vi "Software package Integrity Tool.vi"() -> ()   [LabVIEW 2010]
uses:
  SIT_Data.ctl
  package/VIE.Module.Queued Message Handler.enqueue.State.PolyChild.QueuedMessageHandler.vi
  package/VIE.Module.Queued Message Handler.[enqueue].State.PolyChild.QueuedMessageHandler.vi
  <vilib>/Utility/config.llb/Read Key (String).vi
  package/Remove Duplicates from 1D Array (Path)__ogtk.vi
  package/VIE.Module.Queued Message Handler.QueuedMessageHandler.dqGOOPClass.lvlib
  <vilib>/Utility/config.llb/NI_LVConfig.lvlib
panel:
  out "File list not ok":string
  out "Package not ok":bool
  in  "Color Box":u32(colorbox)
  out "File List 2":i32[](listbox)
  out "Active Row:Cell Background Color":u32
  in  "chk package integrity":bool
  out "Error Out":errorcluster
  in  "Exit":bool
  in  "Add Package Integrity File":bool
  in  "Delete Package Integrity File":bool
  in  "Package Integrity Files":i32(listbox)
  in  "System Integrity File Path":path
  in  "Save System Integrity File":bool
  in  "User Name":string
  in  "Purpose":string
  in  "Package Revision":string
  in  "Package ID":string
  in  "Package Integrity File Path":path
  in  "Undo":bool
  in  "Save Package Integrity File":bool
  in  "Remove Selected Files":bool
  in  "Add VI Hierarchy":bool
  in  "Recursive":bool
  in  "Add Directory":bool
  in  "Add File":bool
  out "Selection Log":string
  in  "File List":i32[](listbox)
  in  "error in (no error)":errorcluster
  out "error out":errorcluster
  out "CVT (out)":T1
  # "Use the CVT as a data bus for data that is\nto be accesed outside of the VI.  It can be\nused for data passed around  inside the state\nmachine too, and all local data can be selectively\npurged from the CVT in the \"system.Exit\" state."
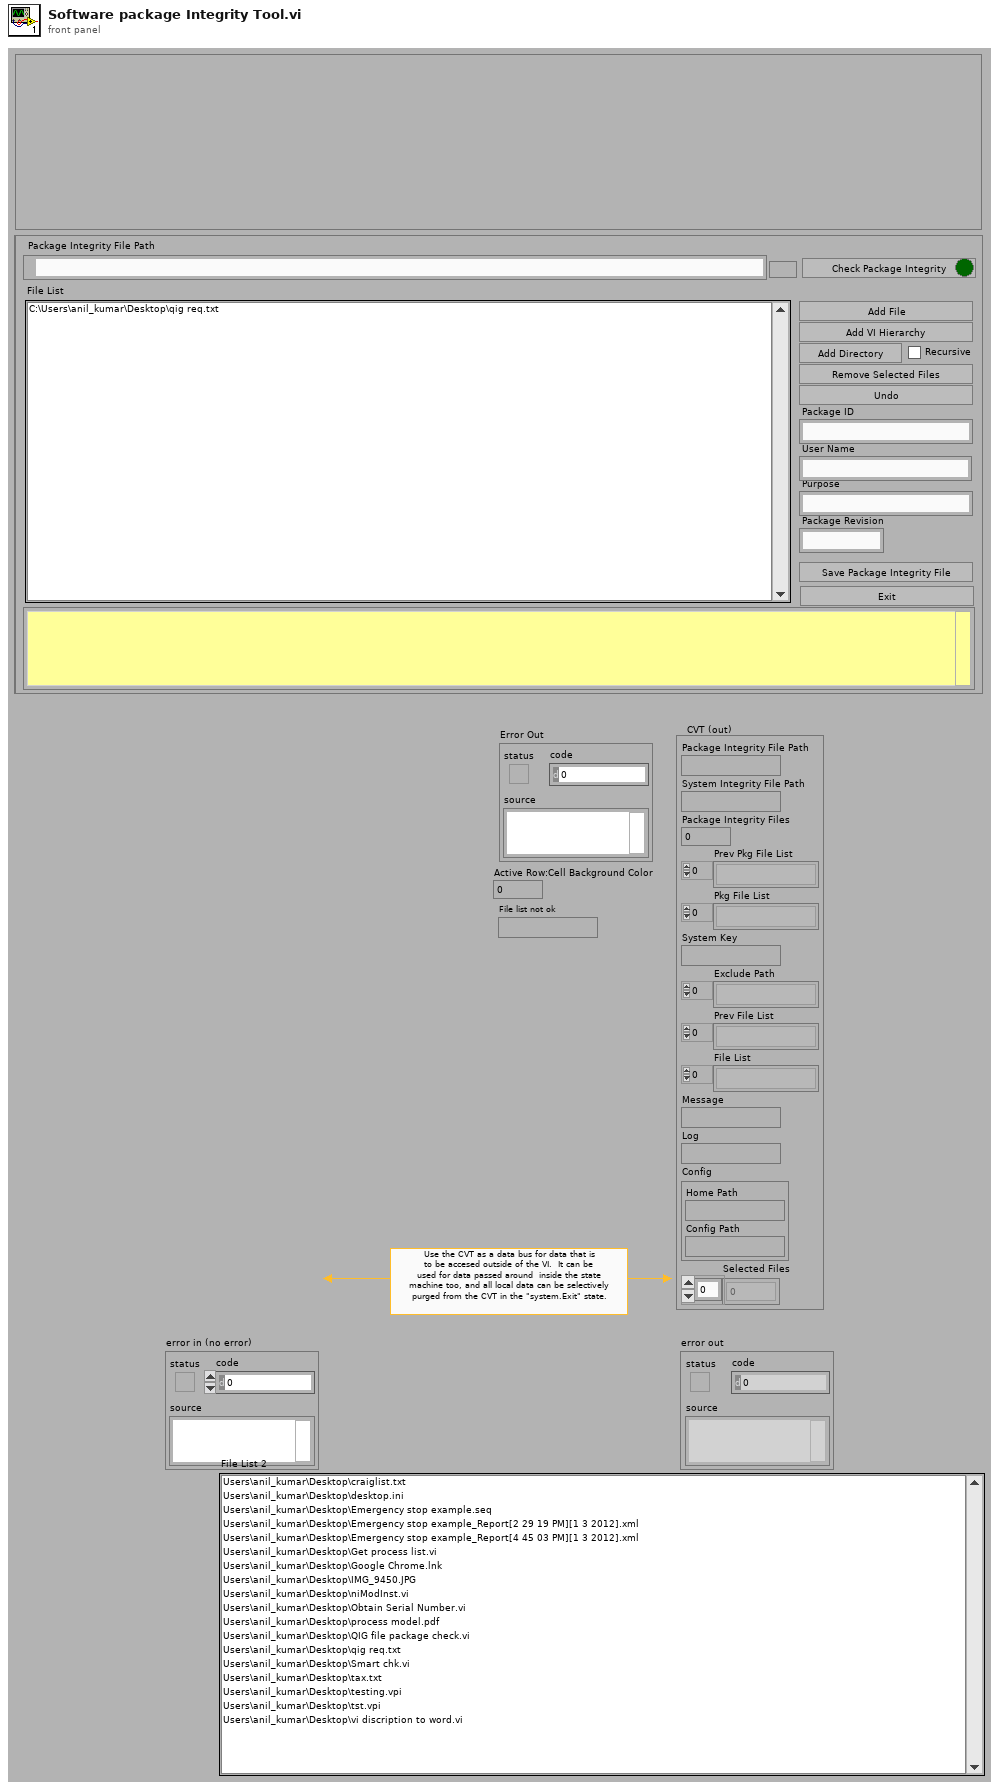
[diagram p1: front panel]
types:
  T1 = typedef "SIT_Data.ctl" = cluster{"Package Integrity File Path":path, "System Integrity File Path":path, "Package Integrity Files":i32, "Prev Pkg File List":path[], "Pkg File List":path[], "System Key":string, "Exclude Path":path[], "Prev File List":path[], "File List":path[], "Message":string, "Log":string, "Config":cluster{"Home Path":path, "Config Path":path}, "Selected Files":i32[]}
  T2 = typedef "VIE.Module.Queued Message Handler.QueuedMessageHandler.dqGOOPClass.lvlib/VIE.Module.Queued Message Handler.dqClass_ObjectReference.ctl" = refnum<k1>
  T3 = typedef "NI_LVConfig.lvlib/Config Data RefNum.ctl" = refnum<k1>
  T4 = enum32{"existing file", "new file", "new or existing file", "existing dir", "new dir", "new or existing dir", "existing file (use LLBs)", "new file (use LLBs)", "new or existing file (use LLBs)", "new or existing file or directory (use LLBs)", "existing dir (use LLBs)", "new dir (use LLBs)", "new or existing dir (use LLBs)", "existing file or dir", "new file or dir", "new or existing file or dir", "existing file or dir (use LLBs)", "new file or dir (use LLBs)"}
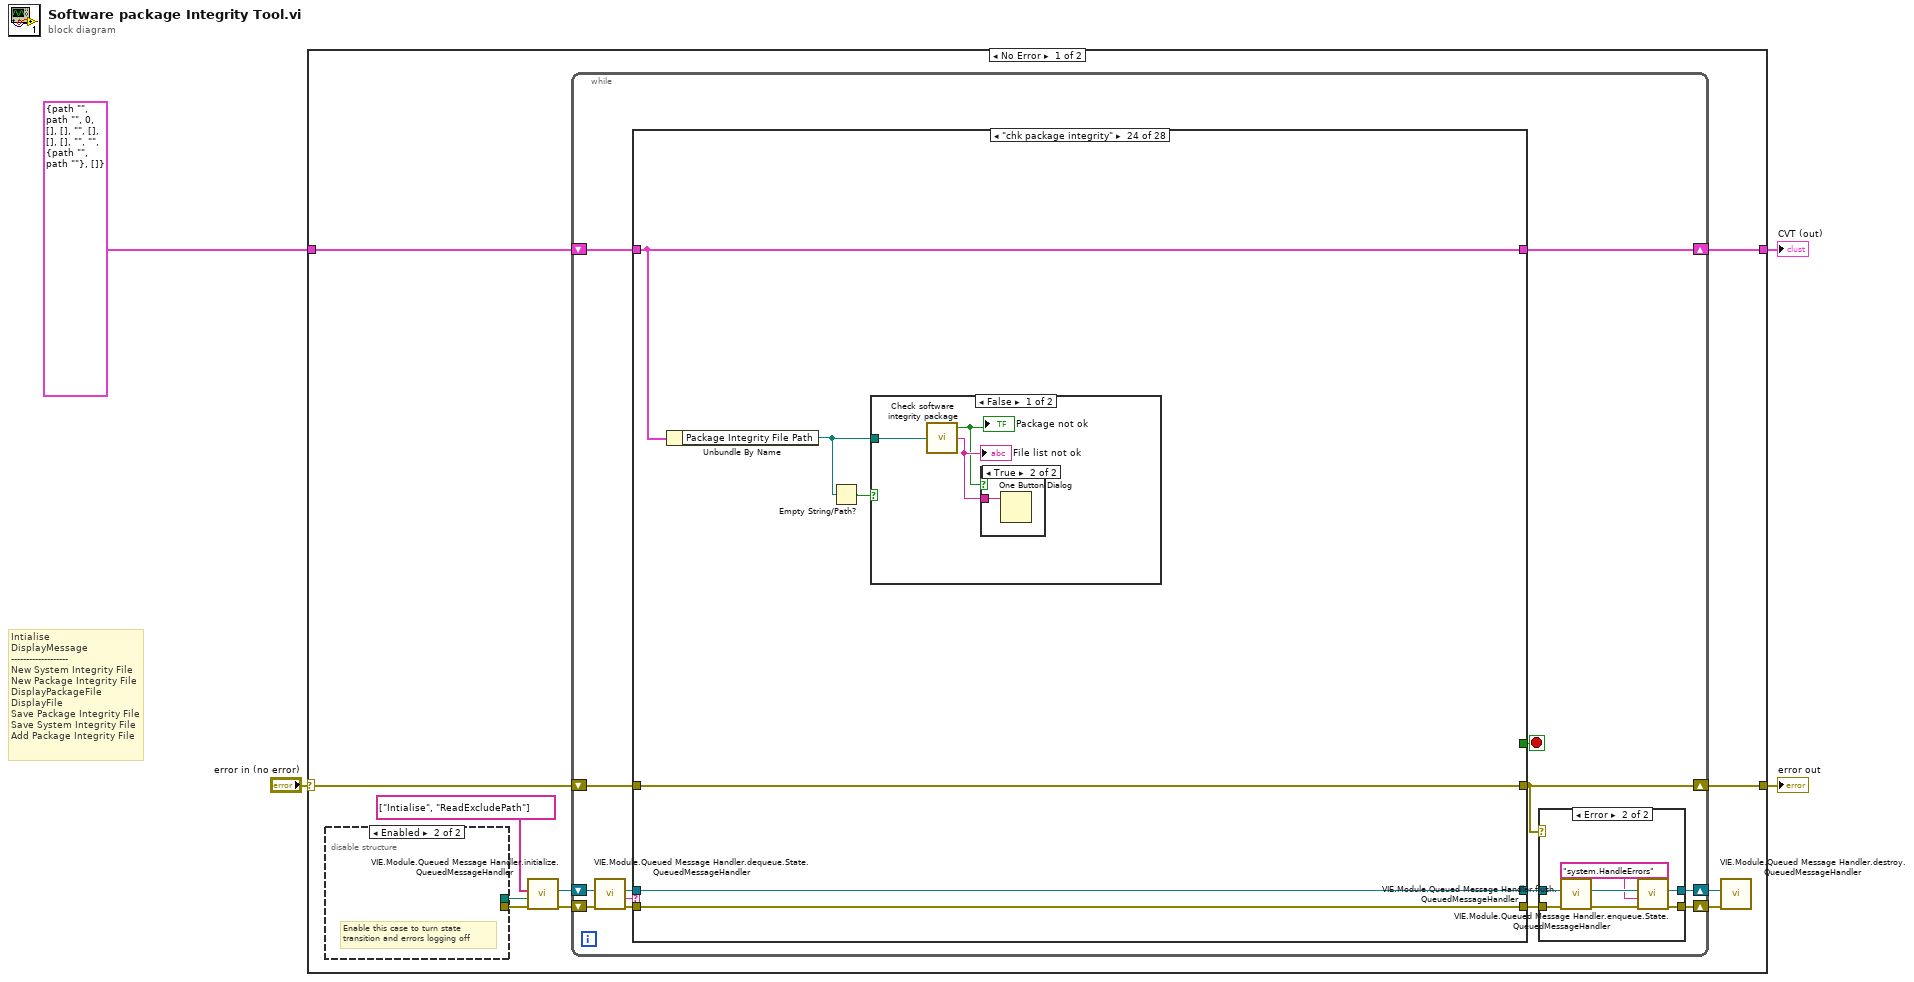
[diagram p0: block diagram]
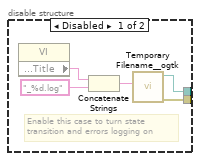
[diagram p2: hidden frame]
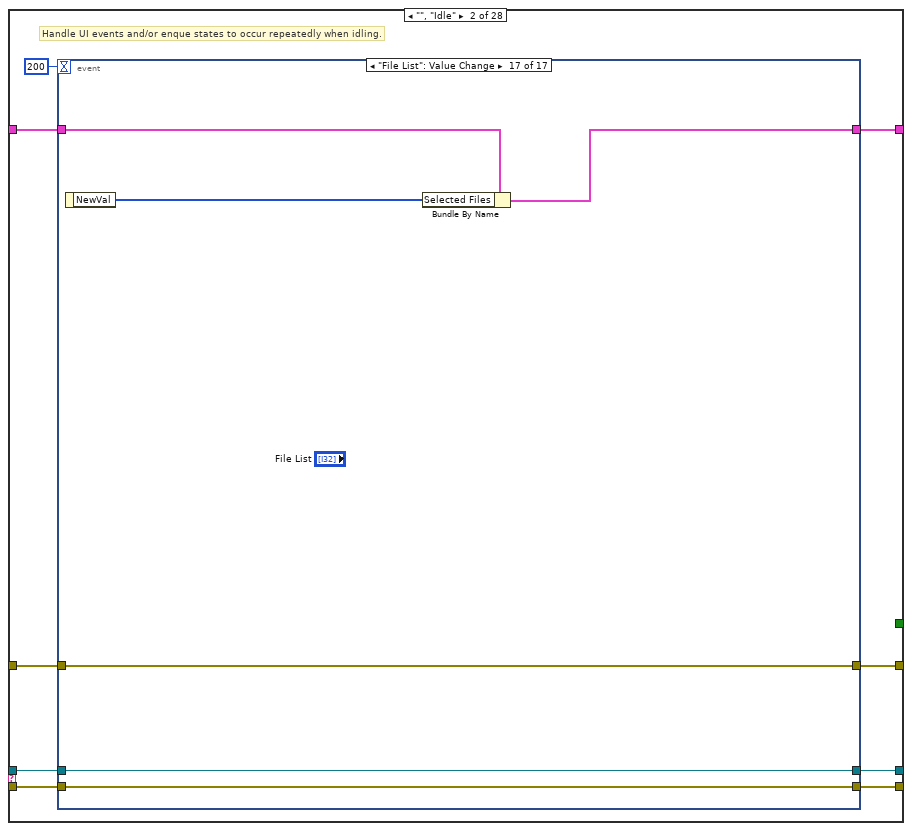
[diagram p5: hidden frame]
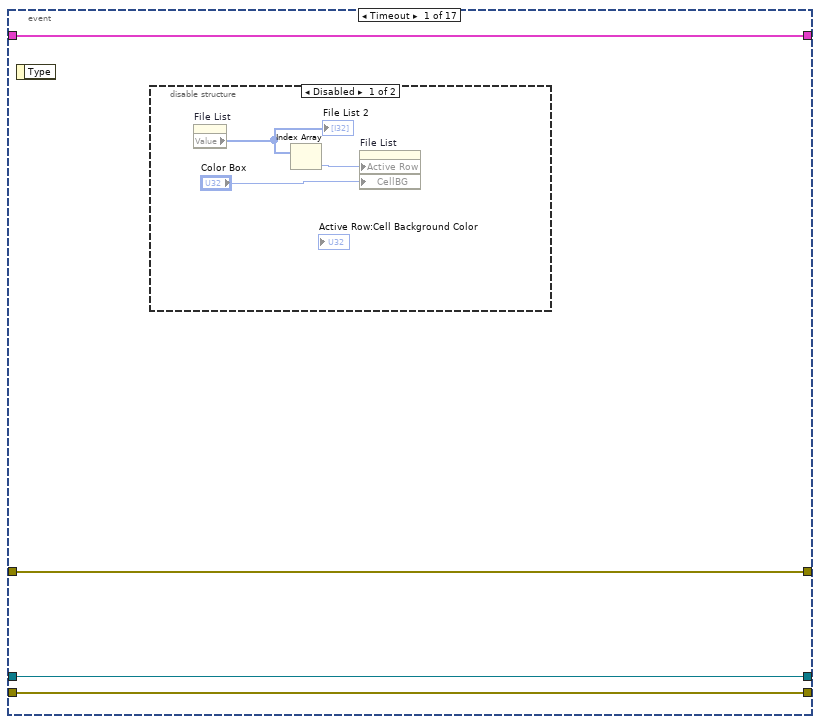
[diagram p6: hidden frame]
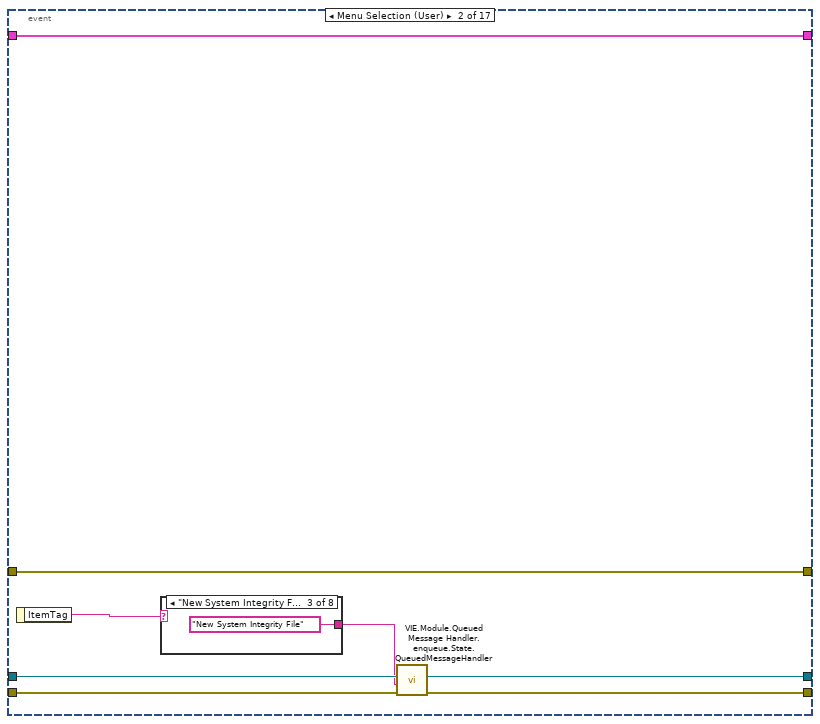
[diagram p8: hidden frame]
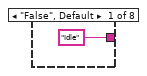
[diagram p9: hidden frame]
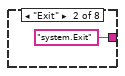
[diagram p10: hidden frame]
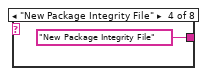
[diagram p11: hidden frame]
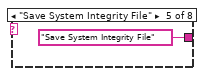
[diagram p12: hidden frame]
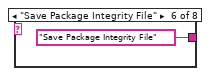
[diagram p13: hidden frame]
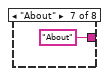
[diagram p14: hidden frame]
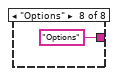
[diagram p15: hidden frame]
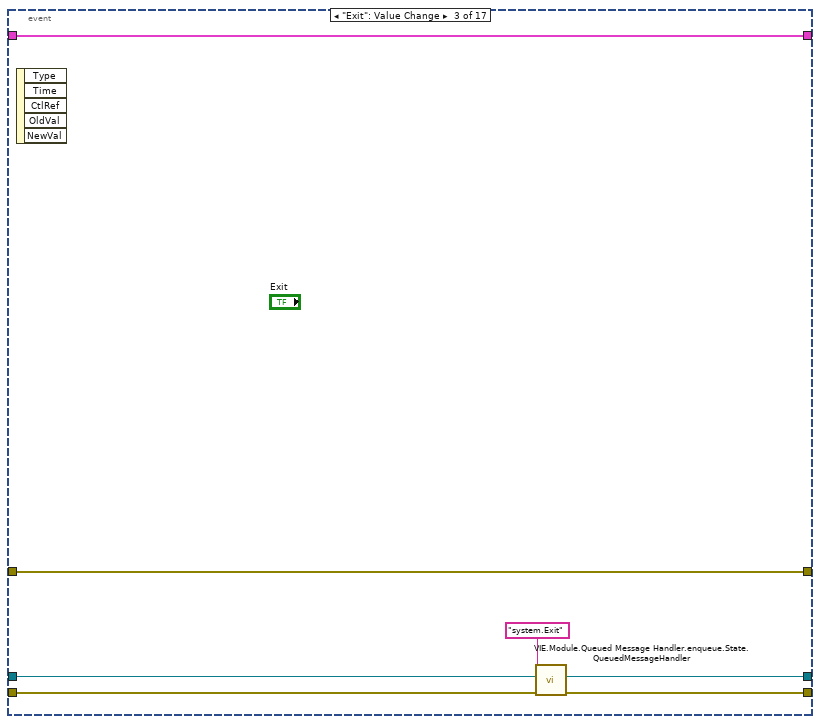
[diagram p16: hidden frame]
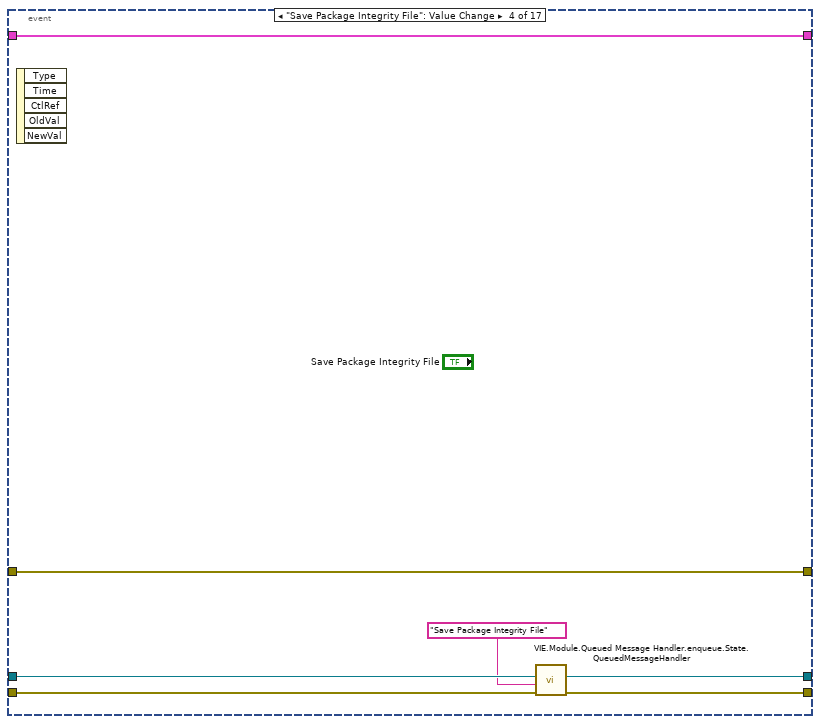
[diagram p17: hidden frame]
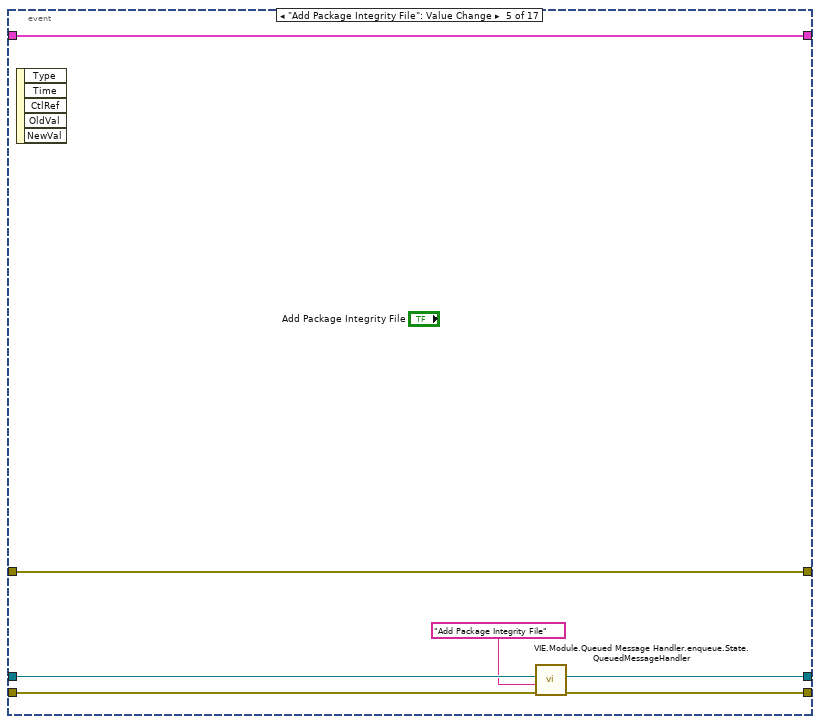
[diagram p18: hidden frame]
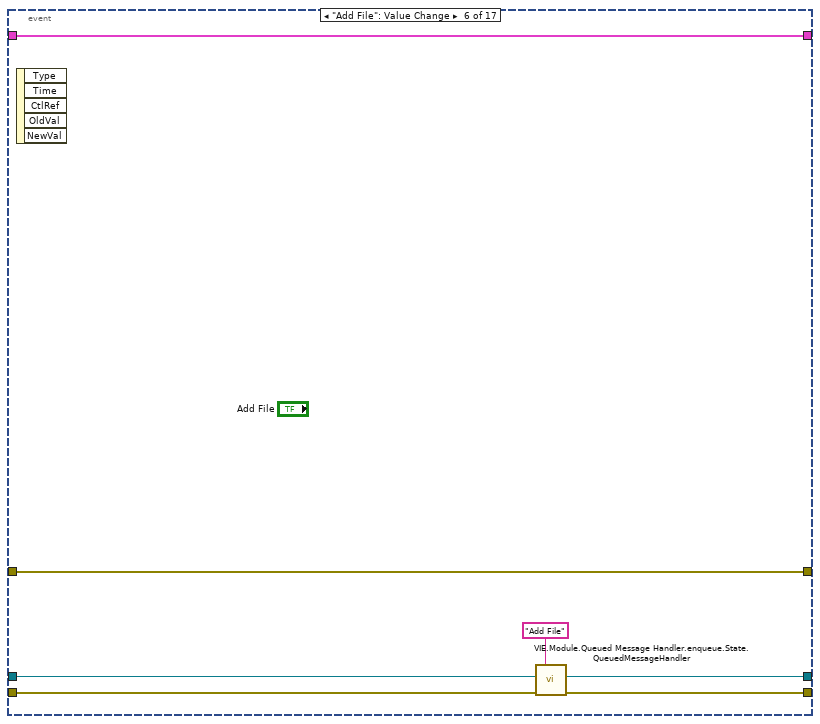
[diagram p19: hidden frame]
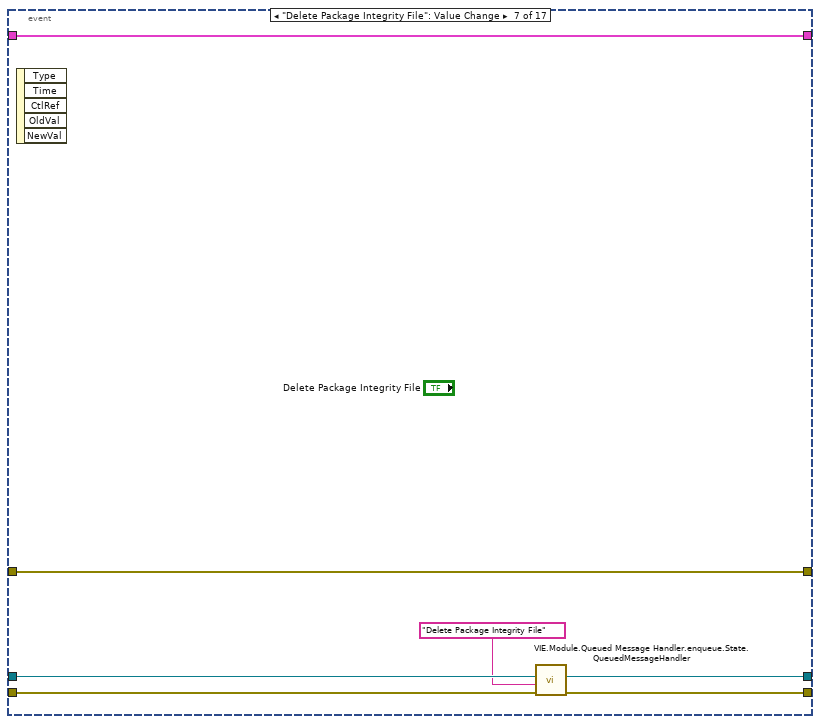
[diagram p20: hidden frame]
diagram:
  # "Intialise\nDisplayMessage\n-------------------\nNew System Integrity File\nNew Package Integrity File\nDisplayPackageFile\nDisplayFile\nSave Package Integrity File\nSave System Integrity File\nAdd Package Integrity File"
  n1 = case shown="No Error" "error in (no error)" {
    selector: "error in (no error)" -> [w8 w754]
    tunnel: [w7 w754] -> w2
    tunnel: T1 {"Package Integrity File Path"=path "", "System Integrity File Path"=path "", "Package Integrity Files"=0, "Prev Pkg File List"=[], "Pkg File List"=[], "System Key"="", "Exclude Path"=[], "Prev File List"=[], "File List"=[], "Message"="", "Log"="", "Config"={"Home Path"=path "", "Config Path"=path ""}, "Selected Files"=[]} ("CVT (in)") -> [w5 w753]
    tunnel: [w9 w753] -> w4
    frame No Error {
      n2 = disable-structure shown="Enabled" {
        disable-tunnel: [w17 _] -> w11
        disable-tunnel: [w16 _] -> w10
        frame Disabled {
          # "Enable this case to turn state\ntransition and errors logging on"
          n3 = property class="VI"() -> ("Front Panel.Title"=w18:string)  [unwired: 2 in, 2 out]
          n4 = Concatenate Strings(w18, "_%d.log" ("string")) -> (w20:string)
          n5 = call <userlib>:"Temporary Filename__ogtk.vi"("pattern (lvtemp%d.tmp)"=w20) -> ("error out"=w17:errorcluster, "file in tmp dir"=w16:path)  [unwired: 5 in]
        }
        frame Enabled {
          # "Enable this case to turn state\ntransition and errors logging off"
        }
      }
      n6 = call "VIE.Module.Queued Message Handler.initialize.QueuedMessageHandler.vi"("error in (no error)"=w11, "State Queue Log FilePath (\"\" = Do Not Log)"=w10, "Initial State Queue (empty)"=string[] ["Intialise", "ReadExcludePath"] ("Initial State Queue")) -> ("error out"=w15:errorcluster, "QueuedMessageHandler.dqGOOPClass (out)"=w12:T2)  [unwired: 7 in]
      n7 = while {
        shift-right: [w23] -> w14
        shift-left: w15 -> [w31]
        shift-right: [w28] -> w9
        shift-left: w5 -> [w29]
        shift-right: [w26] -> w7
        shift-left: w8 -> [w27]
        shift-right: [w22] -> w13
        shift-left: w12 -> [w34]
        stop <- w21 stop-if-true
        n8 = call "VIE.Module.Queued Message Handler.dequeue.State.QueuedMessageHandler.vi"("error in (no error)"=w31, "QueuedMessageHandler.dqGOOPClass (in)"=w34) -> ("error out"=w32:errorcluster, "State Dequeued"=w30:string, "QueuedMessageHandler.dqGOOPClass (out)"=w33:T2)  [unwired: 7 in]
        n9 = case shown="\"chk package integrity\"" w30 {
          selector: w30 -> [_ _ _ _ _ _ _ _ _ _ _ _ _ _ _ _ _ _ _ _ _ _ _ _ _ w714 _ _]
          tunnel: w32 -> [w44 w54 w203 w210 w231 w236 w265 w271 w277 w293 w308 w349 w360 w388 w410 w462 w479 w512 w542 w575 w630 w645 w655 w701 w708 w713 w731 w749]
          tunnel: [w44 w49 w200 w210 w231 w235 w263 w270 w277 w291 w306 w347 w359 w387 w409 w461 w478 w511 w541 w574 w629 w644 w654 w701 w708 w713 w722 w749] -> w25
          tunnel: w33 -> [w45 w53 w202 w211 w232 w234 w266 w269 w278 w294 w309 w350 w358 w386 w412 w460 w477 w510 w540 w573 w628 w643 w653 w702 w709 w712 w732 w750]
          tunnel: [w45 w50 w201 w211 w232 w233 w264 w268 w278 w292 w307 w348 w357 w385 w411 w459 w476 w509 w539 w572 w627 w642 w652 w702 w709 w712 w723 w750] -> w24
          tunnel: w29 -> [w47 w56 w207 w213 w222 w242 w267 w274 w280 w287 w300 w339 w366 w391 w419 w453 w471 w504 w536 w569 w626 w641 w659 w700 w711 w721 w735 w748]
          tunnel: [w47 w52 w206 w217 w221 w241 w267 w274 w280 w286 w304 w338 w365 w390 w418 w452 w470 w503 w535 w568 w625 w640 w658 w700 w711 w721 w735 w748] -> w28
          tunnel: w27 -> [w46 w55 w208 w212 w230 w243 w261 w275 w279 w289 w302 w345 w371 w399 w417 _ w469 w502 w534 w567 w624 w639 w674 w703 w710 w716 w733 w751]
          tunnel: [w46 w51 w194 w214 w230 w243 w261 w275 w279 w289 w301 w345 w371 w399 w416 w449 w468 w501 w533 w566 w624 w639 w674 w703 w710 w715 w726 w751] -> w26
          tunnel: [_ _ _ _ _ _ _ _ _ _ _ _ _ _ _ _ _ _ _ _ _ _ _ _ _ _ _ TRUE] -> w21
          frame "---- Custom States --------------------------" {
            # "Do not put any code in here - this is a case divider, and is not a valid state, so any code here will not be executed."
          }
          frame "", "Idle" {
            # "Handle UI events and/or enque states to occur repeatedly when idling."
            n10 = event shown="[16] \"File List\": Value Change" {
              selector: _ -> [_ _ _ _ _ _ _ _ _ _ _ _ _ _ _ _ _]
              dyn-events: _ -> [_ _ _ _ _ _ _ _ _ _ _ _ _ _ _ _ _]
              timeout: 200 -> [_ _ _ _ _ _ _ _ _ _ _ _ _ _ _ _ _]
              tunnel: w56 -> [w60 w71 w86 w93 w100 w107 w114 w121 w128 w135 w142 w149 w152 w162 w171 w185 w189]
              tunnel: w55 -> [w57 w70 w85 w92 w99 w106 w113 w120 w127 w134 w141 w148 w158 w169 w178 w184 w191]
              tunnel: w54 -> [w58 w69 w84 w91 w98 w105 w112 w119 w126 w133 w140 w147 w157 w168 w177 w181 w186]
              tunnel: w53 -> [w59 w67 w82 w89 w96 w103 w110 w117 w124 w131 w138 w145 w155 w166 w175 w182 w187]
              tunnel: [w60 w71 w86 w93 w100 w107 w114 w121 w128 w135 w142 w149 w151 w163 w172 w185 w190] -> w52
              tunnel: [w57 w70 w85 w92 w99 w106 w113 w120 w127 w134 w141 w148 w158 w169 w178 w184 w191] -> w51
              tunnel: [w59 w66 w81 w88 w95 w102 w109 w116 w123 w130 w137 w144 w154 w165 w174 w180 w187] -> w50
              tunnel: [w58 w68 w83 w90 w97 w104 w111 w118 w125 w132 w139 w146 w156 w167 w176 w179 w186] -> w49
              event Timeout {
                n11 = event-data() -> ()  [unwired: 1 in, 1 out]
                n12 = disable-structure shown="Disabled" {
                  frame Disabled {
                    n13 = property on="File List" class="LstBox (strict)"() -> ("Value"=w63:i32[])  [unwired: 2 in, 2 out]
                    "File List 2" <- w63
                    n14 = Index Array(array=w63) -> (element=w62:i32)  [unwired: 1 in]
                    n15 = property on="File List" class="LstBox (strict)"("Active Row"=w62, "CellBG"="Color Box") -> ()  [unwired: 2 in, 2 out]
                  }
                  frame Enabled {
                  }
                }
              }
              event Menu Selection (User) {
                n16 = event-data() -> ("ItemTag"=w65:string)  [unwired: 1 in]
                n17 = case shown="\"New System Integrity File\"" w65 {
                  tunnel: ["Idle" ("ItemTag") "system.Exit" ("ItemTag") "New System Integrity File" ("ItemTag") "New Package Integrity File" ("ItemTag") "Save System Integrity File" ("ItemTag") "Save Package Integrity File" ("ItemTag") "About" ("ItemTag") "Options" ("ItemTag")] -> w64
                  frame "False", Default {
                  }
                  frame "Exit" {
                  }
                  frame "New System Integrity File" {
                  }
                  frame "New Package Integrity File" {
                  }
                  frame "Save System Integrity File" {
                  }
                  frame "Save Package Integrity File" {
                  }
                  frame "About" {
                  }
                  frame "Options" {
                  }
                }
                n18 = call-poly "VIE.Module.Queued Message Handler.enqueue.State.QueuedMessageHandler.vi"("error in (no error)"=w69, "State to Enqueue"=w64, "QueuedMessageHandler.dqGOOPClass (in)"=w67) -> ("error out"=w68:errorcluster, "QueuedMessageHandler.dqGOOPClass (out)"=w66:T2)  [unwired: 7 in]
              }
              event "Exit": Value Change {
                n19 = event-data() -> ()  [unwired: 1 in, 5 out]
                n20 = call-poly "VIE.Module.Queued Message Handler.enqueue.State.QueuedMessageHandler.vi"("error in (no error)"=w84, "State to Enqueue"="system.Exit", "QueuedMessageHandler.dqGOOPClass (in)"=w82) -> ("error out"=w83:errorcluster, "QueuedMessageHandler.dqGOOPClass (out)"=w81:T2)  [unwired: 7 in]
              }
              event "Save Package Integrity File": Value Change {
                n21 = event-data() -> ()  [unwired: 1 in, 5 out]
                n22 = call-poly "VIE.Module.Queued Message Handler.enqueue.State.QueuedMessageHandler.vi"("error in (no error)"=w91, "State to Enqueue"="Save Package Integrity File", "QueuedMessageHandler.dqGOOPClass (in)"=w89) -> ("error out"=w90:errorcluster, "QueuedMessageHandler.dqGOOPClass (out)"=w88:T2)  [unwired: 7 in]
              }
              event "Add Package Integrity File": Value Change {
                n23 = event-data() -> ()  [unwired: 1 in, 5 out]
                n24 = call-poly "VIE.Module.Queued Message Handler.enqueue.State.QueuedMessageHandler.vi"("error in (no error)"=w98, "State to Enqueue"="Add Package Integrity File", "QueuedMessageHandler.dqGOOPClass (in)"=w96) -> ("error out"=w97:errorcluster, "QueuedMessageHandler.dqGOOPClass (out)"=w95:T2)  [unwired: 7 in]
              }
              event "Add File": Value Change {
                n25 = event-data() -> ()  [unwired: 1 in, 5 out]
                n26 = call-poly "VIE.Module.Queued Message Handler.enqueue.State.QueuedMessageHandler.vi"("error in (no error)"=w105, "State to Enqueue"="Add File", "QueuedMessageHandler.dqGOOPClass (in)"=w103) -> ("error out"=w104:errorcluster, "QueuedMessageHandler.dqGOOPClass (out)"=w102:T2)  [unwired: 7 in]
              }
              event "Delete Package Integrity File": Value Change {
                n27 = event-data() -> ()  [unwired: 1 in, 5 out]
                n28 = call-poly "VIE.Module.Queued Message Handler.enqueue.State.QueuedMessageHandler.vi"("error in (no error)"=w112, "State to Enqueue"="Delete Package Integrity File", "QueuedMessageHandler.dqGOOPClass (in)"=w110) -> ("error out"=w111:errorcluster, "QueuedMessageHandler.dqGOOPClass (out)"=w109:T2)  [unwired: 7 in]
              }
              event "Remove Selected Files": Value Change {
                n29 = event-data() -> ()  [unwired: 1 in, 5 out]
                n30 = call-poly "VIE.Module.Queued Message Handler.enqueue.State.QueuedMessageHandler.vi"("error in (no error)"=w119, "State to Enqueue"="Remove Selected Files", "QueuedMessageHandler.dqGOOPClass (in)"=w117) -> ("error out"=w118:errorcluster, "QueuedMessageHandler.dqGOOPClass (out)"=w116:T2)  [unwired: 7 in]
              }
              event "Add Directory": Value Change {
                n31 = event-data() -> ()  [unwired: 1 in, 5 out]
                n32 = call-poly "VIE.Module.Queued Message Handler.enqueue.State.QueuedMessageHandler.vi"("error in (no error)"=w126, "State to Enqueue"="Add Directory", "QueuedMessageHandler.dqGOOPClass (in)"=w124) -> ("error out"=w125:errorcluster, "QueuedMessageHandler.dqGOOPClass (out)"=w123:T2)  [unwired: 7 in]
              }
              event "Add VI Hierarchy": Value Change {
                n33 = event-data() -> ()  [unwired: 1 in, 5 out]
                n34 = call-poly "VIE.Module.Queued Message Handler.enqueue.State.QueuedMessageHandler.vi"("error in (no error)"=w133, "State to Enqueue"="Add VI Hierarchy", "QueuedMessageHandler.dqGOOPClass (in)"=w131) -> ("error out"=w132:errorcluster, "QueuedMessageHandler.dqGOOPClass (out)"=w130:T2)  [unwired: 7 in]
              }
              event "Undo": Value Change {
                n35 = event-data() -> ()  [unwired: 1 in, 5 out]
                n36 = call-poly "VIE.Module.Queued Message Handler.enqueue.State.QueuedMessageHandler.vi"("error in (no error)"=w140, "State to Enqueue"="Undo", "QueuedMessageHandler.dqGOOPClass (in)"=w138) -> ("error out"=w139:errorcluster, "QueuedMessageHandler.dqGOOPClass (out)"=w137:T2)  [unwired: 7 in]
              }
              event "Save System Integrity File": Value Change {
                n37 = event-data() -> ()  [unwired: 1 in, 5 out]
                n38 = call-poly "VIE.Module.Queued Message Handler.enqueue.State.QueuedMessageHandler.vi"("error in (no error)"=w147, "State to Enqueue"="Save System Integrity File", "QueuedMessageHandler.dqGOOPClass (in)"=w145) -> ("error out"=w146:errorcluster, "QueuedMessageHandler.dqGOOPClass (out)"=w144:T2)  [unwired: 7 in]
              }
              event "System Integrity File Path": Value Change {
                n39 = event-data() -> ("NewVal"=w150:path)  [unwired: 1 in]
                n40 = Bundle By Name(cluster=w152, "System Integrity File Path"=w150) -> (w151:T1)
                n41 = call-poly "VIE.Module.Queued Message Handler.enqueue.State.QueuedMessageHandler.vi"("error in (no error)"=w157, "State to Enqueue"="Load System Integrity File", "QueuedMessageHandler.dqGOOPClass (in)"=w155) -> ("error out"=w156:errorcluster, "QueuedMessageHandler.dqGOOPClass (out)"=w154:T2)  [unwired: 7 in]
              }
              event "Package Integrity Files": Value Change {
                n42 = event-data() -> ("NewVal"=w159:i32)  [unwired: 1 in]
                n43 = Unbundle By Name(w162) -> ("Pkg File List"=w161:path[])
                n44 = Index Array(array=w161, index=w159) -> (element=w160:path)
                n45 = local write "Package Integrity File Path"(w160) -> ()
                n46 = Bundle By Name(cluster=w162, "Package Integrity File Path"=w160, "Package Integrity Files"=w159) -> (w163:T1)
                n47 = call-poly "VIE.Module.Queued Message Handler.enqueue.State.QueuedMessageHandler.vi"("error in (no error)"=w168, "State to Enqueue"="Load Package Integrity File", "QueuedMessageHandler.dqGOOPClass (in)"=w166) -> ("error out"=w167:errorcluster, "QueuedMessageHandler.dqGOOPClass (out)"=w165:T2)  [unwired: 7 in]
              }
              event "Package Integrity File Path": Value Change {
                n48 = event-data() -> ()  [unwired: 1 in, 1 out]
                n49 = Bundle By Name(cluster=w171, "Package Integrity File Path"="Package Integrity File Path") -> (w172:T1)
                n50 = call-poly "VIE.Module.Queued Message Handler.enqueue.State.QueuedMessageHandler.vi"("error in (no error)"=w177, "State to Enqueue"="Load Package Integrity File", "QueuedMessageHandler.dqGOOPClass (in)"=w175) -> ("error out"=w176:errorcluster, "QueuedMessageHandler.dqGOOPClass (out)"=w174:T2)  [unwired: 7 in]
              }
              event "chk package integrity": Value Change {
                n51 = event-data() -> ()  [unwired: 1 in, 1 out]
                n52 = call-poly "VIE.Module.Queued Message Handler.enqueue.State.QueuedMessageHandler.vi"("error in (no error)"=w181, "State to Enqueue"="chk package integrity", "QueuedMessageHandler.dqGOOPClass (in)"=w182) -> ("error out"=w179:errorcluster, "QueuedMessageHandler.dqGOOPClass (out)"=w180:T2)  [unwired: 7 in]
              }
              event "File List": Value Change {
                n53 = event-data() -> ("NewVal"=w188:i32[])  [unwired: 1 in]
                n54 = Bundle By Name(cluster=w189, "Selected Files"=w188) -> (w190:T1)
              }
            }
          }
          frame "Intialise" {
            w195 = path "" ("Package Integrity File Path")
            w196 = string[] [] ("Item Names")
            n55 = call "Fit VI window to Largest Dec__ogtk.vi"("error in (no error)"=w208) -> ("error out"=w194:errorcluster)  [unwired: 5 in, 1 out]
            n56 = Current VI's Path() -> (path=w198:path)
            n57 = Strip Path(path=w198) -> (stripped path=w197:path)  [unwired: 1 out]
            n58 = Build Path(base path=w197, name or relative path="System Integrity Tool setting.ini") -> (appended path=w193:path)
            n59 = local write "System Integrity File Path"(w195) -> ()
            n60 = local write "Package not ok"(FALSE ("Package file ok")) -> ()
            n61 = local write "Package Integrity File Path"(w195) -> ()
            n62 = Bundle By Name(cluster=w207, "Message"="Welcome to the Package Integrity File Generation Utility, brought to you by VI Engineering, Inc." ("queue element"), "Config.Home Path"=w197, "Config.Config Path"=w193) -> (w206:T1)
            n63 = property on="Package Integrity Files" class="LstBox (strict)"("Item Names"=w196) -> ()  [unwired: 2 in, 2 out]
            n64 = property on="File List" class="LstBox (strict)"("Item Names"=w196) -> ()  [unwired: 2 in, 2 out]
            n65 = call-poly "VIE.Module.Queued Message Handler.enqueue.State.QueuedMessageHandler.vi"("error in (no error)"=w203, "State to Enqueue"="DisplayMessage", "QueuedMessageHandler.dqGOOPClass (in)"=w202) -> ("error out"=w200:errorcluster, "QueuedMessageHandler.dqGOOPClass (out)"=w201:T2)  [unwired: 7 in]
          }
          frame "ReadExcludePath" {
            n66 = Unbundle By Name(w213) -> ("Config.Config Path"=w209:path)
            n67 = call "Read Write Exclude path.vi"("path In"=w209, "Error In"=w212) -> ("Key out"=w216:string, "Exclude Path Out"=w215:path[], "Error Out"=w214:errorcluster)  [unwired: 10 in, 1 out]
            n68 = Bundle By Name(cluster=w213, "System Key"=w216, "Exclude Path"=w215) -> (w217:T1)
          }
          frame "DisplayMessage" {
            n69 = Unbundle By Name(w222) -> ("Log"=w225:string, "Message"=w219:string)
            n70 = Empty String/Path?(string/path=w219) -> (empty?=w229:bool)
            n71 = Select(t="", s=w229, f="\r") -> (s? t:f=w227:string)
            n72 = Concatenate Strings(w225, w227, w219) -> (w224:string)
            n73 = call "SIT_Limit Display.vi"("Limit"=100 ("Number of Lines"), "Data In"=w224) -> ("Line Count"=w218:i32, "Data Out"=w220:string)  [unwired: 8 in]
            "Selection Log" <- w220
            n74 = property on="Selection Log" class="Str"("Text.Scroll Position"=w218) -> ()  [unwired: 2 in, 2 out]
            n75 = Bundle By Name(cluster=w222, "Log"=w220) -> (w221:T1)
          }
          frame "Undo" {
            n76 = Unbundle By Name(w242) -> ("Prev File List"=w239:path[], "File List"=w238:path[])
            n77 = disable-structure shown="Disabled" {
              disable-tunnel: [w246 ""] -> w240
              disable-tunnel: w239 -> [w245 _]
              disable-tunnel: w238 -> [w244 _]
              frame Disabled {
                n78 = Array Size(array=w245) -> (size(s)=w248:i32)
                n79 = Array Size(array=w244) -> (size(s)=w247:i32)
                n80 = Greater?(x=w248, y=w247) -> (0:w249:bool)
                n81 = case shown="True" w249 {
                  tunnel: w248 -> [w252 w258]
                  tunnel: w247 -> [w251 w257]
                  tunnel: [w250 w255] -> w246
                  frame False {
                    n82 = Subtract(x=w251, y=w252) -> (x-y=w254:i32)
                    n83 = Format Into String(format string="Undo: %d File(s) Removed from List" ("Format String"), w254) -> (resulting string=w250:string)  [unwired: 2 in, 1 out]
                  }
                  frame True {
                    n84 = Subtract(x=w258, y=w257) -> (x-y=w256:i32)
                    n85 = Format Into String(format string="Undo: %d File(s) Added Back to List" ("Format String"), w256) -> (resulting string=w255:string)  [unwired: 2 in, 1 out]
                  }
                }
              }
              frame Enabled {
              }
            }
            n86 = call-poly "VIE.Module.Queued Message Handler.enqueue.State.QueuedMessageHandler.vi"("error in (no error)"=w236, "States to Enqueue"=string[] ["DisplayMessage", "DisplayFile"], "QueuedMessageHandler.dqGOOPClass (in)"=w234) -> ("error out"=w235:errorcluster, "QueuedMessageHandler.dqGOOPClass (out)"=w233:T2)  [unwired: 7 in]
            n87 = Bundle By Name(cluster=w242, "File List"=w239, "Prev File List"=w238, "Message"=w240) -> (w241:T1)
          }
          frame "custom.CleanUp" {
            n88 = call-poly "VIE.Module.Queued Message Handler.enqueue.State.QueuedMessageHandler.vi"("error in (no error)"=w265, "State to Enqueue"="system.Exit", "QueuedMessageHandler.dqGOOPClass (in)"=w266) -> ("error out"=w263:errorcluster, "QueuedMessageHandler.dqGOOPClass (out)"=w264:T2)  [unwired: 7 in]
          }
          frame "Options" {
            n89 = Unbundle By Name(w274) -> ("Config.Config Path"=w273:path)
            n90 = call "Exclude Path Options.vi"("Error In"=w275, "Path In"=w273) -> ()  [unwired: 9 in, 1 out]
            n91 = call-poly "VIE.Module.Queued Message Handler.enqueue.State.QueuedMessageHandler.vi"("error in (no error)"=w271, "State to Enqueue"="ReadExcludePath", "QueuedMessageHandler.dqGOOPClass (in)"=w269) -> ("error out"=w270:errorcluster, "QueuedMessageHandler.dqGOOPClass (out)"=w268:T2)  [unwired: 7 in]
          }
          frame "About" {
            n92 = One Button Dialog(message="Purpose of this tool is for System Integrity") -> ()  [unwired: 1 in, 1 out]
          }
          frame "Load Package Integrity File" {
            n93 = Unbundle By Name(w287) -> ("Package Integrity File Path"=w288:path)
            n94 = call "Load Package Config.vi"("Path"=w288) -> ("Path Out"=w285:path[], "Package ID"=w284:string, "Purpose"=w283:string, "Package Revision"=w282:string, "Error Out"=→"Error Out":errorcluster)  [unwired: 9 in, 1 out]
            n95 = local write "Purpose"(w283) -> ()
            n96 = local write "Package ID"(w284) -> ()
            n97 = local write "Package Revision"(w282) -> ()
            n98 = call-poly "VIE.Module.Queued Message Handler.enqueue.State.QueuedMessageHandler.vi"("error in (no error)"=w293, "State to Enqueue"="DisplayFile", "QueuedMessageHandler.dqGOOPClass (in)"=w294) -> ("error out"=w291:errorcluster, "QueuedMessageHandler.dqGOOPClass (out)"=w292:T2)  [unwired: 7 in]
            n99 = Bundle By Name(cluster=w287, "Prev File List"=w285, "File List"=w285) -> (w286:T1)
          }
          frame "Load System Integrity File" {
            n100 = Unbundle By Name(w300) -> ("System Integrity File Path"=w299:path)
            n101 = call <vilib>:"Open Config Data.vi"("error in (no error)"=w302, "create file if necessary (T)"=FALSE, "configuration file path"=w299) -> ("error out"=w295:errorcluster, "refnum"=w303:T3)  [unwired: 6 in, 1 out]
            n102 = case shown="No Error" w295 {
              selector: w295 -> [w310 _]
              tunnel: w303 -> [w315 _]
              tunnel: [w314 _] -> w301
              tunnel: [w313 _] -> w298
              frame No Error {
                w321 = "Package Integrity Files" ("section")
                n103 = call <vilib>:"Get Key Names.vi"("section"=w321, "error in (no error)"=w310, "refnum"=w315) -> ("error out"=w320:errorcluster, "key names"=w322:string[], "refnum out"=w319:T3)  [unwired: 5 in, 1 out]
                n104 = for {
                  tunnel: w322 -> [w331] mode=indexing
                  tunnel: w321 -> [w330]
                  tunnel: w320 -> [w329]
                  tunnel: [w328] -> w318
                  tunnel: w319 -> [w327]
                  tunnel: [w326] -> w317
                  tunnel: [w324] -> w316 mode=indexing
                  n105 = call-poly <vilib>:"Read Key.vi"("section"=w330, "error in (no error)"=w329, "default value"="", "key"=w331, "refnum"=w327) -> ("error out"=w328:errorcluster, "value"=w324:string, "refnum out"=w326:T3)  [unwired: 3 in, 1 out]
                }
                n106 = call <vilib>:"Close Config Data.vi"("error in (no error)"=w318, "write file if changed (T)"=FALSE, "refnum"=w317) -> ("error out"=w314:errorcluster, "file path"=w312:path)  [unwired: 7 in]
                n107 = Strip Path(path=w312) -> (stripped path=w311:path)  [unwired: 1 out]
                n108 = for "Extract File Paths" {
                  tunnel: w316 -> [w335] mode=indexing
                  tunnel: [w333] -> w313 mode=indexing
                  tunnel: w311 -> [w332]
                  n109 = String To Path(string=w335) -> (path=w334:path)
                  n110 = call "Rel to Abs Path.vi"("Rel File Path"=w334, "Base Path"=w332) -> ("Path Out"=w333:path)  [unwired: 8 in, 1 out]
                }
              }
              frame Error {
              }
            }
            n111 = call-poly "VIE.Module.Queued Message Handler.enqueue.State.QueuedMessageHandler.vi"("error in (no error)"=w308, "State to Enqueue"="DisplayFile", "QueuedMessageHandler.dqGOOPClass (in)"=w309) -> ("error out"=w306:errorcluster, "QueuedMessageHandler.dqGOOPClass (out)"=w307:T2)  [unwired: 7 in]
            n112 = Index Array(array=w298) -> (element=w297:path)  [unwired: 1 in]
            n113 = Bundle By Name(cluster=w300, "Prev Pkg File List"=w298, "Pkg File List"=w298, "Package Integrity File Path"=w297) -> (w304:T1)
          }
          frame "New System Integrity File" {
            (unwired) T4."new file" ("select mode (2)")
            n114 = Unbundle By Name(w339) -> ("System Integrity File Path"=w340:path)
            n115 = Strip Path(path=w340) -> (stripped path=w344:path)  [unwired: 1 out]
            n116 = File Dialog(6:"*.vsi" ("pattern"), 7:"New System Integrity File" ("prompt"), 11:w344) -> (0:w341:errorcluster, 1:w336:bool, 3:w337:path)  [unwired: 4 in, 1 out]
            n117 = case shown="False" w336 {
              tunnel: w341 -> [_ _]
              tunnel: w339 -> [w355 w356]
              tunnel: [w354 w356] -> w338
              tunnel: w337 -> [w352 _]
              frame False {
                w353 = path[] []
                n118 = Bundle By Name(cluster=w355, "Prev Pkg File List"=w353, "Pkg File List"=w353, "System Integrity File Path"=w352) -> (w354:T1)
                n119 = property on="Package Integrity Files" class="LstBox (strict)"("Value"=-1 ("Package Integrity Files")) -> ()  [unwired: 2 in, 2 out]
                n120 = local write "System Integrity File Path"(w352) -> ()
              }
              frame True {
              }
            }
            n121 = call-poly "VIE.Module.Queued Message Handler.enqueue.State.QueuedMessageHandler.vi"("error in (no error)"=w349, "State to Enqueue"="DisplayPackageFile", "QueuedMessageHandler.dqGOOPClass (in)"=w350) -> ("error out"=w347:errorcluster, "QueuedMessageHandler.dqGOOPClass (out)"=w348:T2)  [unwired: 7 in]
          }
          frame "New Package Integrity File" {
            n122 = Unbundle By Name(w366) -> ("System Integrity File Path"=w367:path)
            n123 = Strip Path(path=w367) -> (stripped path=w370:path)  [unwired: 1 out]
            n124 = File Dialog(6:"*.vpi" ("pattern"), 7:"New Package Integrity File" ("prompt"), 11:w370) -> (0:w362:errorcluster, 1:w363:bool, 3:w364:path)  [unwired: 4 in, 1 out]
            n125 = case shown="False" w363 {
              tunnel: w366 -> [w375 w381]
              tunnel: [w374 w381] -> w365
              tunnel: w364 -> [w373 _]
              tunnel: w362 -> [_ _]
              frame False {
                w372 = path[] [] ("Prev File List")
                n126 = Strip Path(path=w373) -> (name=w379:string)  [unwired: 1 out]
                n127 = local write "Package Integrity File Path"(w373) -> ()
                n128 = Bundle By Name(cluster=w375, "File List"=w372, "Prev File List"=w372, "Package Integrity File Path"=w373) -> (w374:T1)
                n129 = property on="Package Integrity Files" class="LstBox (strict)"("Value"=-1 ("Package Integrity Files")) -> ()  [unwired: 2 in, 2 out]
                n130 = Match Pattern(string=w379, regular expression=".vpi$") -> (before substring=w376:string)  [unwired: 1 in, 3 out]
                n131 = local write "Package Revision"("") -> ()
                n132 = local write "Package ID"(w376) -> ()
              }
              frame True {
              }
            }
            n133 = call-poly "VIE.Module.Queued Message Handler.enqueue.State.QueuedMessageHandler.vi"("error in (no error)"=w360, "State to Enqueue"="DisplayFile", "QueuedMessageHandler.dqGOOPClass (in)"=w358) -> ("error out"=w359:errorcluster, "QueuedMessageHandler.dqGOOPClass (out)"=w357:T2)  [unwired: 7 in]
          }
          frame "DisplayPackageFile" {
            # "Message Queue"
            n134 = Unbundle By Name(w391) -> ("System Integrity File Path"=w392:path, "Pkg File List"=w384:path[])
            n135 = call-poly "Remove Duplicates from 1D Array__ogtk.vi"("Input Array"=w384) -> ("Output Array"=w398:path[])  [unwired: 1 out]
            n136 = Strip Path(path=w392) -> (stripped path=w393:path)  [unwired: 1 out]
            n137 = Sort 1D Array(array=w398) -> (sorted array=w382:path[])
            n138 = Array Size(array=w384) -> (size(s)=w396:i32)
            n139 = Array Size(array=w382) -> (size(s)=w395:i32)
            n140 = Not Equal?(x=w396, y=w395) -> (x != y?=w397:bool)
            n141 = case shown="True" w397 {
              tunnel: w396 -> [_ w407]
              tunnel: w395 -> [_ w408]
              tunnel: [_ w404] -> w383
              frame False {
              }
              frame True {
                n142 = Subtract(x=w407, y=w408) -> (x-y=w405:i32)
                n143 = Format Into String(format string="    %d Repeated File(s) Found and Removed from System Integrity File list" ("Format String"), w405) -> (resulting string=w404:string)  [unwired: 2 in, 1 out]
              }
            }
            n144 = for {
              tunnel: w393 -> [w403]
              tunnel: w382 -> [w402] mode=indexing
              tunnel: [w400] -> w394 mode=indexing
              n145 = call "Abs to Rel Path.vi"("File Path"=w402, "Base Path"=w403) -> ("Path Out"=w401:path)  [unwired: 8 in, 1 out]
              n146 = Path To String(path=w401) -> (string=w400:string)
            }
            n147 = call-poly "VIE.Module.Queued Message Handler.enqueue.State.QueuedMessageHandler.vi"("error in (no error)"=w388, "States to Enqueue"=string[] ["DisplayMessage"], "QueuedMessageHandler.dqGOOPClass (in)"=w386) -> ("error out"=w387:errorcluster, "QueuedMessageHandler.dqGOOPClass (out)"=w385:T2)  [unwired: 7 in]
            n148 = property on="Package Integrity Files" class="LstBox (strict)"("Item Names"=w394) -> ()  [unwired: 2 in, 2 out]
            n149 = Bundle By Name(cluster=w391, "Pkg File List"=w382, "Message"=w383) -> (w390:T1)
          }
          frame "Save Package Integrity File" {
            n150 = Unbundle By Name(w419) -> ("Package Integrity File Path"=w415:path, "File List"=w414:path[], "System Key"=w420:string)
            n151 = Empty Array?(array=w414) -> (empty?=w413:bool)
            n152 = case shown="False" w413 {
              tunnel: w420 -> [w439 _]
              tunnel: w419 -> [w438 w445]
              tunnel: [w437 w445] -> w418
              tunnel: w417 -> [w436 w448]
              tunnel: [w435 w448] -> w416
              tunnel: w415 -> [w423 _]
              tunnel: w414 -> [w434 _]
              tunnel: w412 -> [w427 w447]
              tunnel: [w426 w447] -> w411
              tunnel: w410 -> [w425 w446]
              tunnel: [w424 w446] -> w409
              frame False {
                n153 = Empty String/Path?(string/path=w423) -> (empty?=w422:bool)
                n154 = case shown="False" w422 {
                  tunnel: [w440 w441] -> w421
                  tunnel: w423 -> [w440 _]
                  frame False {
                  }
                  frame True {
                    n155 = File Dialog(6:"*.vpi" ("pattern (all files)")) -> (3:w441:path)  [unwired: 6 in, 3 out]
                  }
                }
                n156 = call "Generate Package Integrity File.vi"("PackageID"="Package ID", "PackageRev"="Package Revision", "Purpose"="Purpose", "System Key"=w439, "USER_NAME"="User Name", "Error In"=w436, "Package File Paths"=w434, "Integrity File Path"=w421) -> ("error out"=w435:errorcluster)  [unwired: 11 in]
                n157 = local write "Package Integrity File Path"(w421) -> ()
                n158 = case shown="Error" w435 {
                  tunnel: ["Create Package Integrity File...Done..." ("Message") "Error in creating file" ("Message")] -> w429
                  frame No Error {
                  }
                  frame Error {
                  }
                }
                n159 = call-poly "VIE.Module.Queued Message Handler.enqueue.State.QueuedMessageHandler.vi"("error in (no error)"=w425, "States to Enqueue"=string[] ["DisplayMessage"], "QueuedMessageHandler.dqGOOPClass (in)"=w427) -> ("error out"=w424:errorcluster, "QueuedMessageHandler.dqGOOPClass (out)"=w426:T2)  [unwired: 7 in]
                n160 = Bundle By Name(cluster=w438, "Package Integrity File Path"=w421, "Message"=w429) -> (w437:T1)
              }
              frame True {
              }
            }
          }
          frame "Save System Integrity File" {
            n161 = Unbundle By Name(w453) -> ("System Integrity File Path"=w458:path, "Pkg File List"=w457:path[], "System Key"=w456:string)
            n162 = local read "User Name"() -> (w455:string)
            n163 = call "Generate System Integrity File.vi"("System Integrity File Path"=w458, "File Paths"=w457, "System Key"=w456, "USER_NAME"=w455) -> ("Error Out"=w449:errorcluster)  [unwired: 15 in]
            n164 = case shown="Error" w449 {
              tunnel: ["Done..." ("Message") "There was an error creating the System Integrity File" ("queue element")] -> w450
              frame No Error {
              }
              frame Error {
              }
            }
            n165 = call-poly "VIE.Module.Queued Message Handler.enqueue.State.QueuedMessageHandler.vi"("error in (no error)"=w462, "States to Enqueue"=string[] ["DisplayMessage"], "QueuedMessageHandler.dqGOOPClass (in)"=w460) -> ("error out"=w461:errorcluster, "QueuedMessageHandler.dqGOOPClass (out)"=w459:T2)  [unwired: 7 in]
            n166 = Concatenate Strings("Create System Integrity File....." ("Message"), w450) -> (w451:string)
            n167 = Bundle By Name(cluster=w453, "Message"=w451) -> (w452:T1)
          }
          frame "Add File" {
            n168 = Unbundle By Name(w471) -> ("File List"=w466:path[], "Package Integrity File Path"=w474:path)
            n169 = Strip Path(path=w474) -> (stripped path=w475:path)  [unwired: 1 out]
            n170 = File Dialog(11:w475) -> (0:w472:errorcluster, 1:w473:bool, 3:w467:path)  [unwired: 6 in, 1 out]
            n171 = case shown="False" w473 {
              tunnel: w479 -> [w492 w495]
              tunnel: [w491 w495] -> w478
              tunnel: w477 -> [w490 w496]
              tunnel: [w489 w496] -> w476
              tunnel: w472 -> [_ _]
              tunnel: w471 -> [w488 w497]
              tunnel: [w487 w497] -> w470
              tunnel: [w486 w494] -> w468
              tunnel: w469 -> [w486 w494]
              tunnel: w467 -> [w484 _]
              tunnel: w466 -> [w485 _]
              frame False {
                n172 = Path To String(path=w484) -> (string=w482:string)
                n173 = Build Array (concatenate)(w485, w484) -> (w483:path[])
                n174 = Concatenate Strings("Added File: " ("Message"), w482) -> (w481:string)
                n175 = call-poly "VIE.Module.Queued Message Handler.enqueue.State.QueuedMessageHandler.vi"("error in (no error)"=w492, "States to Enqueue"=string[] ["DisplayMessage", "DisplayFile"], "QueuedMessageHandler.dqGOOPClass (in)"=w490) -> ("error out"=w491:errorcluster, "QueuedMessageHandler.dqGOOPClass (out)"=w489:T2)  [unwired: 7 in]
                n176 = Bundle By Name(cluster=w488, "Prev File List"=w485, "File List"=w483, "Message"=w481) -> (w487:T1)
              }
              frame True {
              }
            }
          }
          frame "Add Package Integrity File" {
            n177 = Unbundle By Name(w504) -> ("Pkg File List"=w499:path[], "System Integrity File Path"=w507:path)
            n178 = Strip Path(path=w507) -> (stripped path=w508:path)  [unwired: 1 out]
            n179 = File Dialog(6:"*.vpi" ("pattern (all files)"), 11:w508) -> (0:w505:errorcluster, 1:w506:bool, 3:w500:path)  [unwired: 5 in, 1 out]
            n180 = case shown="False" w506 {
              tunnel: w512 -> [w525 w528]
              tunnel: [w524 w528] -> w511
              tunnel: w510 -> [w523 w529]
              tunnel: [w522 w529] -> w509
              tunnel: w505 -> [_ _]
              tunnel: w504 -> [w521 w530]
              tunnel: [w520 w530] -> w503
              tunnel: [w519 w527] -> w501
              tunnel: w502 -> [w519 w527]
              tunnel: w500 -> [w517 _]
              tunnel: w499 -> [w518 _]
              frame False {
                n181 = Path To String(path=w517) -> (string=w515:string)
                n182 = Build Array (concatenate)(w518, w517) -> (w516:path[])
                n183 = Concatenate Strings("Added Package Integrity File: " ("Message"), w515) -> (w514:string)
                n184 = call-poly "VIE.Module.Queued Message Handler.enqueue.State.QueuedMessageHandler.vi"("error in (no error)"=w525, "States to Enqueue"=string[] ["DisplayMessage", "DisplayPackageFile"], "QueuedMessageHandler.dqGOOPClass (in)"=w523) -> ("error out"=w524:errorcluster, "QueuedMessageHandler.dqGOOPClass (out)"=w522:T2)  [unwired: 7 in]
                n185 = Bundle By Name(cluster=w521, "Prev Pkg File List"=w518, "Pkg File List"=w516, "Message"=w514) -> (w520:T1)
              }
              frame True {
              }
            }
          }
          frame "Add Directory" {
            n186 = Unbundle By Name(w536) -> ("File List"=w531:path[])
            n187 = File Dialog() -> (0:w537:errorcluster, 1:w538:bool, 3:w532:path)  [unwired: 7 in, 1 out]
            n188 = case shown="False" w538 {
              tunnel: w542 -> [w557 w560]
              tunnel: [w556 w560] -> w541
              tunnel: w540 -> [w555 w561]
              tunnel: [w554 w561] -> w539
              tunnel: w537 -> [_ _]
              tunnel: w536 -> [w553 w562]
              tunnel: [w552 w562] -> w535
              tunnel: [w551 w559] -> w533
              tunnel: w534 -> [w551 w559]
              tunnel: w532 -> [w548 _]
              tunnel: w531 -> [w550 _]
              frame False {
                n189 = call "Get Recursive File details.vi"("Recursive?"="Recursive", "Path"=w548) -> ("Count"=w545:i32, "File Details"=w547:path[])  [unwired: 8 in]
                n190 = Build Array (concatenate)(w550, w547) -> (w549:path[])
                n191 = Format Into String(format string="Added %d File: " ("Message"), w545) -> (resulting string=w543:string)  [unwired: 2 in, 1 out]
                n192 = call-poly "VIE.Module.Queued Message Handler.enqueue.State.QueuedMessageHandler.vi"("error in (no error)"=w557, "States to Enqueue"=string[] ["DisplayMessage", "DisplayFile"], "QueuedMessageHandler.dqGOOPClass (in)"=w555) -> ("error out"=w556:errorcluster, "QueuedMessageHandler.dqGOOPClass (out)"=w554:T2)  [unwired: 7 in]
                n193 = Bundle By Name(cluster=w553, "Prev File List"=w550, "File List"=w549, "Message"=w543) -> (w552:T1)
              }
              frame True {
              }
            }
          }
          frame "Add VI Hierarchy" {
            n194 = Unbundle By Name(w569) -> ("File List"=w564:path[])
            n195 = File Dialog(6:"*.vi" ("pattern")) -> (0:w570:errorcluster, 1:w571:bool, 3:w565:path)  [unwired: 6 in, 1 out]
            n196 = case shown="False" w571 {
              tunnel: w575 -> [w590 w613]
              tunnel: [w589 w613] -> w574
              tunnel: w573 -> [w588 w614]
              tunnel: [w587 w614] -> w572
              tunnel: w570 -> [_ _]
              tunnel: w569 -> [w586 w615]
              tunnel: [w585 w615] -> w568
              tunnel: [w584 w612] -> w566
              tunnel: w567 -> [w584 w612]
              tunnel: w565 -> [w578 _]
              tunnel: w564 -> [w583 _]
              frame False {
                n197 = Strip Path(path=w578) -> (name=w582:string)  [unwired: 1 out]
                n198 = Match Pattern(string=w582, regular expression=".[Vv][Ii]$") -> (offset past match=w580:i32)  [unwired: 1 in, 3 out]
                n199 = Path To String(path=w578) -> (string=w577:string)
                n200 = case shown="0, Default" w580 {
                  tunnel: w578 -> [w608 w611]
                  tunnel: [w609 w610] -> w579
                  tunnel: [w606 _] -> w576
                  frame 0, Default {
                    n201 = Build Array(w608) -> (w607:path[])
                    n202 = call "Get VI Hierarchy Lists.vi"("Top-level VI Paths"=w607) -> ("List of VIs"=w609:path[], "error out"=w606:errorcluster)  [unwired: 11 in, 2 out]
                  }
                  frame -1 {
                    n203 = Build Array(w611) -> (w610:path[])
                  }
                }
                n204 = case shown="No Error" w576 {
                  tunnel: w586 -> [w600 w605]
                  tunnel: [w599 w604] -> w585
                  tunnel: w583 -> [w598 _]
                  tunnel: w579 -> [w594 _]
                  tunnel: w577 -> [w592 w603]
                  frame No Error {
                    n205 = Array Size(array=w594) -> (size(s)=w593:i32)
                    n206 = Build Array (concatenate)(w598, w594) -> (w597:path[])
                    n207 = Format Into String(format string="Added Hierarchy %s\nAdded %d File: " ("Message"), w592, w593) -> (resulting string=w595:string)  [unwired: 2 in, 1 out]
                    n208 = Bundle By Name(cluster=w600, "Prev File List"=w598, "File List"=w597, "Message"=w595) -> (w599:T1)
                  }
                  frame Error {
                    n209 = Concatenate Strings("Error in Adding Vi Hierarchy :" ("Message"), w603) -> (w601:string)
                    n210 = Bundle By Name(cluster=w605, "Message"=w601) -> (w604:T1)
                  }
                }
                n211 = call-poly "VIE.Module.Queued Message Handler.enqueue.State.QueuedMessageHandler.vi"("error in (no error)"=w590, "States to Enqueue"=string[] ["DisplayMessage", "DisplayFile"], "QueuedMessageHandler.dqGOOPClass (in)"=w588) -> ("error out"=w589:errorcluster, "QueuedMessageHandler.dqGOOPClass (out)"=w587:T2)  [unwired: 7 in]
              }
              frame True {
              }
            }
          }
          frame "Delete Package Integrity File" {
            n212 = Unbundle By Name(w626) -> ("Pkg File List"=w617:path[], "Package Integrity Files"=w616:i32)
            n213 = Delete From Array(array=w617, index=w616) -> (deleted portion=w619:path, array with subset deleted=w618:path[])  [unwired: 1 in]
            n214 = Path To String(path=w619) -> (string=w622:string)
            n215 = Concatenate Strings("Deleted Package Integrity File: " ("Message"), w622) -> (w620:string)
            n216 = call-poly "VIE.Module.Queued Message Handler.enqueue.State.QueuedMessageHandler.vi"("error in (no error)"=w630, "States to Enqueue"=string[] ["DisplayMessage", "DisplayPackageFile"], "QueuedMessageHandler.dqGOOPClass (in)"=w628) -> ("error out"=w629:errorcluster, "QueuedMessageHandler.dqGOOPClass (out)"=w627:T2)  [unwired: 7 in]
            n217 = Bundle By Name(cluster=w626, "Prev Pkg File List"=w617, "Pkg File List"=w618, "Message"=w620) -> (w625:T1)
          }
          frame "Remove Selected Files" {
            n218 = Unbundle By Name(w641) -> ("File List"=w636:path[], "Selected Files"=w632:i32[])
            n219 = Reverse 1D Array(array=w632) -> (reversed array=w634:i32[])
            n220 = for {
              tunnel: w634 -> [w646] mode=indexing
              shift-right: [w648] -> w637
              shift-left: w636 -> [w647]
              n221 = Delete From Array(array=w647, index=w646) -> (array with subset deleted=w648:path[])  [unwired: 1 in, 1 out]
            }
            n222 = Array Size(array=w632) -> (size(s)=w631:i32)
            n223 = Format Into String(format string="Deleted  %d Files" ("Message"), w631) -> (resulting string=w633:string)  [unwired: 2 in, 1 out]
            n224 = Bundle By Name(cluster=w641, "Prev File List"=w636, "File List"=w637, "Message"=w633) -> (w640:T1)
            n225 = call-poly "VIE.Module.Queued Message Handler.enqueue.State.QueuedMessageHandler.vi"("error in (no error)"=w645, "States to Enqueue"=string[] ["DisplayMessage", "DisplayFile"], "QueuedMessageHandler.dqGOOPClass (in)"=w643) -> ("error out"=w644:errorcluster, "QueuedMessageHandler.dqGOOPClass (out)"=w642:T2)  [unwired: 7 in]
          }
          frame "DisplayFile" {
            # "Message Queue"
            # "Message Queue"
            # "Original List"
            n226 = Unbundle By Name(w659) -> ("File List"=w662:path[], "Exclude Path"=w664:path[], "Package Integrity File Path"=w663:path)
            n227 = call-poly "Remove Duplicates from 1D Array__ogtk.vi"("Input Array"=w662) -> ("Output Array"=w673:path[])  [unwired: 1 out]
            n228 = Sort 1D Array(array=w673) -> (sorted array=w660:path[])
            n229 = for {
              tunnel: w660 -> [w692] mode=indexing
              tunnel: w664 -> [w691]
              tunnel: [w689] -> w661 mode=indexing
              n230 = call "In Any Exclude Path.vi"("Exclude Paths"=w691, "VI Path"=w692) -> ("In Any Exclude Path?"=w690:bool)  [unwired: 9 in]
              n231 = Not(x=w690) -> (.not. x?=w689:bool)
            }
            n232 = Strip Path(path=w663) -> (stripped path=w665:path)  [unwired: 1 out]
            n233 = Array Size(array=w662) -> (size(s)=w671:i32)
            n234 = Array Size(array=w660) -> (size(s)=w670:i32)
            n235 = Not Equal?(x=w671, y=w670) -> (x != y?=w672:bool)
            n236 = call "Select Element from Array.vi"("Data In"=w660, "Select?"=w661) -> ("Data Out"=w657:path[])  [unwired: 13 in]
            n237 = case shown="True" w672 {
              tunnel: w671 -> [_ w696]
              tunnel: w670 -> [_ w697]
              tunnel: [_ w693] -> w651
              frame False {
              }
              frame True {
                n238 = Subtract(x=w696, y=w697) -> (x-y=w694:i32)
                n239 = Format Into String(format string="    %d Repeated File(s) Found and Removed from List" ("Format String"), w694) -> (resulting string=w693:string)  [unwired: 2 in, 1 out]
              }
            }
            n240 = Array Size(array=w660) -> (size(s)=w668:i32)
            n241 = Array Size(array=w657) -> (size(s)=w667:i32)
            n242 = disable-structure shown="Enabled" {
              disable-tunnel: [w677 w683] -> w669
              disable-tunnel: w665 -> [w676 _]
              disable-tunnel: w657 -> [w675 w682]
              frame Disabled {
                n243 = for {
                  tunnel: w676 -> [w681]
                  tunnel: w675 -> [w680] mode=indexing
                  tunnel: [w678] -> w677 mode=indexing
                  n244 = call "Abs to Rel Path.vi"("File Path"=w680, "Base Path"=w681) -> ("Path Out"=w679:path)  [unwired: 8 in, 1 out]
                  n245 = Path To String(path=w679) -> (string=w678:string)
                }
              }
              frame Enabled {
                n246 = Path To String(path=w682) -> (string=w683:string[])
              }
            }
            n247 = Not Equal?(x=w668, y=w667) -> (x != y?=w666:bool)
            n248 = case shown="True" w666 {
              tunnel: w668 -> [_ w687]
              tunnel: w667 -> [_ w688]
              tunnel: [_ w684] -> w650
              frame False {
              }
              frame True {
                n249 = Subtract(x=w687, y=w688) -> (x-y=w685:i32)
                n250 = Format Into String(format string="    %d File(s) In Exclude Paths, therefore Removed" ("Format String"), w685) -> (resulting string=w684:string)  [unwired: 2 in, 1 out]
              }
            }
            n251 = call-poly "VIE.Module.Queued Message Handler.enqueue.State.QueuedMessageHandler.vi"("error in (no error)"=w655, "States to Enqueue"=string[] ["DisplayMessage", "DisplayPackageFile"], "QueuedMessageHandler.dqGOOPClass (in)"=w653) -> ("error out"=w654:errorcluster, "QueuedMessageHandler.dqGOOPClass (out)"=w652:T2)  [unwired: 7 in]
            n252 = property on="File List" class="LstBox (strict)"("Item Names"=w669) -> ()  [unwired: 2 in, 2 out]
            n253 = Concatenate Strings(w650, w651) -> (w649:string)
            n254 = Bundle By Name(cluster=w659, "File List"=w657, "Message"=w649) -> (w658:T1)
          }
          frame "chk package integrity" {
            n255 = Unbundle By Name(w700) -> ("Package Integrity File Path"=w699:path)
            n256 = Empty String/Path?(string/path=w699) -> (empty?=w698:bool)
            n257 = case shown="False" w698 {
              tunnel: w699 -> [w706 _]
              frame False {
                n258 = call "Check software integrity package.vi"("Package Integrity File Path"=w706) -> ("File list not ok"=w705:string, "Package not ok"=w704:bool)  [unwired: 1 in]
                "Package not ok" <- w704
                "File list not ok" <- w705
                n259 = case shown="True" w704 {
                  tunnel: w705 -> [_ w707]
                  frame False {
                  }
                  frame True {
                    n260 = One Button Dialog(message=w707) -> ()  [unwired: 1 in, 1 out]
                  }
                }
              }
              frame True {
              }
            }
          }
          frame "---- System States --------------------------" {
            # "Do not put any code in here - this is a case divider, and is not a valid state, so any code here will not be executed."
          }
          frame "system.StateNameSyntaxError", Default {
            # "Do not alter the code in here - this is a system state that is required by the state machine architecture."
            n261 = property class="VI"() -> ("Name"=w717:string)  [unwired: 2 in, 2 out]
            n262 = Format Into String(format string="Syntax Error - Requested State not found in State Machine Architecture.\n\nArchitecture: %s\nState Requested: %s", w717, w714) -> (resulting string=w718:string)  [unwired: 2 in, 1 out]
            n263 = call <vilib>:"Error Cluster From Error Code.vi"("error in (no error)"=w716, "error message (\"\")"=w718, "error code (0)"=46) -> ("error out"=w715:errorcluster)  [unwired: 6 in]
          }
          frame "system.HandleErrors" {
            # "Do not alter the code in here - this is a system state that is required by the state machine architecture."
            # "Handle errors by presenting a dialog box to the\nuser and logging the error to file (if enabled)"
            n264 = call <vilib>:"Simple Error Handler.vi"("error in (no error)"=w733) -> ("code out"=w729:i32, "source out"=w728:string, "error out"=w730:errorcluster)  [unwired: 4 in, 2 out]
            n265 = Format Into String(format string="ERROR: Code=%d, Source=\"%s\"", w729, w728) -> (resulting string=w727:string)  [unwired: 2 in, 1 out]
            n266 = call <vilib>:"Clear Errors.vi"("error in (no error)"=w730) -> ("error out"=w726:errorcluster)  [unwired: 6 in]
            n267 = call "VIE.Module.Queued Message Handler.logEvent.QueuedMessageHandler.vi"("error in (no error)"=w731, "Event to Log"=w727, "QueuedMessageHandler.dqGOOPClass (in)"=w732) -> ("error out"=w724:errorcluster, "QueuedMessageHandler.dqGOOPClass (out)"=w725:T2)  [unwired: 7 in]
            n268 = disable-structure shown="Enabled" {
              disable-tunnel: w725 -> [w740 w745 w746]
              disable-tunnel: w724 -> [w739 w744 w747]
              disable-tunnel: [w738 w743 w746] -> w723
              disable-tunnel: [w737 w742 w747] -> w722
              frame Disabled {
                # "Enable this case to force software\nto exit on error."
                n269 = call-poly "VIE.Module.Queued Message Handler.enqueue.State.QueuedMessageHandler.vi"("error in (no error)"=w739, "State to Enqueue"="system.Exit", "QueuedMessageHandler.dqGOOPClass (in)"=w740) -> ("error out"=w737:errorcluster, "QueuedMessageHandler.dqGOOPClass (out)"=w738:T2)  [unwired: 7 in]
              }
              frame Disabled {
                # "Enable this case to force software\nto cleanup then exit on error."
                n270 = call-poly "VIE.Module.Queued Message Handler.enqueue.State.QueuedMessageHandler.vi"("error in (no error)"=w744, "States to Enqueue"=string[] ["custom.CleanUp", "system.Exit"], "QueuedMessageHandler.dqGOOPClass (in)"=w745) -> ("error out"=w742:errorcluster, "QueuedMessageHandler.dqGOOPClass (out)"=w743:T2)  [unwired: 7 in]
              }
              frame Enabled {
                # "Enable this case to force software\nto continue on error."
              }
            }
          }
          frame "system.Exit" {
            # "Enable this case to leave all local data added in this VI in the CVT to be\npassed out to the calling VI"
            # "Do not alter the code in here - this is a system state that is required by the state machine architecture."
          }
        }
        n271 = case shown="Error" w26 {
          tunnel: w25 -> [w35 w41]
          tunnel: w24 -> [w36 w40]
          tunnel: [w35 w39] -> w23
          tunnel: [w36 w38] -> w22
          frame No Error {
          }
          frame Error {
            n272 = call "VIE.Module.Queued Message Handler.flush.QueuedMessageHandler.vi"("error in (no error)"=w41, "QueuedMessageHandler.dqGOOPClass (in)"=w40) -> ("error out"=w43:errorcluster, "QueuedMessageHandler.dqGOOPClass (out)"=w42:T2)  [unwired: 7 in, 1 out]
            n273 = call-poly "VIE.Module.Queued Message Handler.enqueue.State.QueuedMessageHandler.vi"("error in (no error)"=w43, "State to Enqueue"="system.HandleErrors", "QueuedMessageHandler.dqGOOPClass (in)"=w42) -> ("error out"=w39:errorcluster, "QueuedMessageHandler.dqGOOPClass (out)"=w38:T2)  [unwired: 7 in]
          }
        }
      }
      n274 = call "VIE.Module.Queued Message Handler.destroy.QueuedMessageHandler.vi"("error in (no error)"=w14, "QueuedMessageHandler.dqGOOPClass (in)"=w13) -> ()  [unwired: 9 in, 1 out]
    }
    frame Error {
      # "An error was passed into the VI, so do not execute and pass the error and input CVT out."
    }
  }
  "error out" <- w2
  "CVT (out)" <- w4
